vi "ke237_setbias_auto.vi"(10 "GPIB address":string="16", 11 "source level":dbl format="%.2f") -> ()   [LabVIEW 2018]
panel:
  in  "error in":T1
  out "error out":T1
  # "Bias range is \"Auto\" and DC delay is \"0\"\n\nSee Ke237 Manual Page 3-19\n\nMZ 4/21/2015"
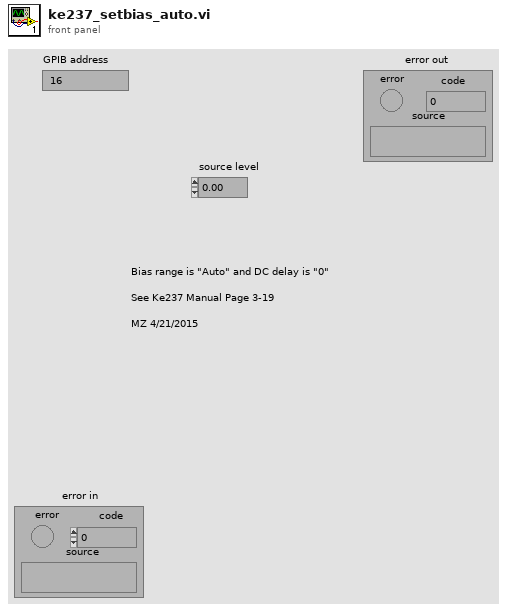
[diagram p1: front panel]
types:
  T1 = cluster{"error":bool, "code":i32, "source":string}
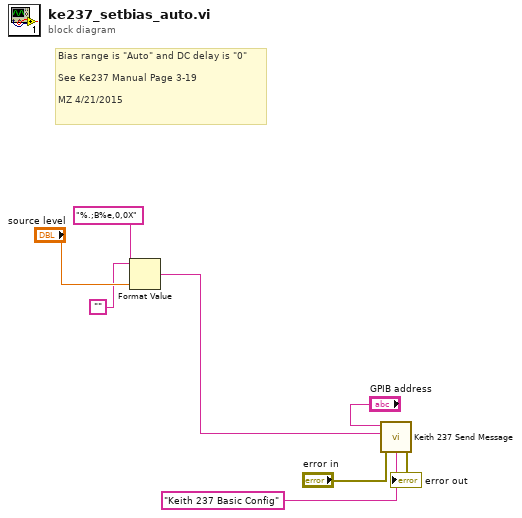
[diagram p0: block diagram]
diagram:
  # "Bias range is \"Auto\" and DC delay is \"0\"\n\nSee Ke237 Manual Page 3-19\n\nMZ 4/21/2015"
  n1 = Format Value(string ("")="", format string="%.;B%e,0,0X", value (0)="source level") -> (output string=w1:string)
  n2 = call <instrlib>:"Keith 237 Send Message.vi"("address string"="GPIB address", "write buffer"=w1, "source"="Keith 237 Basic Config", "error in"="error in") -> ("error out"=→"error out":T1)  [unwired: 2 in, 3 out]
